vi "send_fpga_config_if_not_imgrid (SubVI).vi"(8 "config_trig":dbl[](array[numeric]) format="%0.2f", 9 "img_cluster":cluster{"Take Pic?":bool, "Only Images":bool}, 10 "file_path_cluster":T2, 11 "channel_settings":T1) -> (3 "Only Images":bool)   [LabVIEW 2022 SP3]
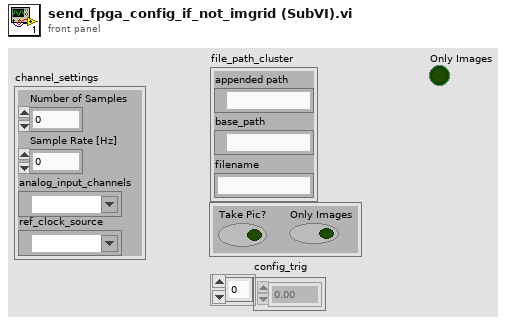
[diagram p1: front panel]
types:
  T1 = cluster{"Number of Samples":i32, "Sample Rate [Hz]":dbl, "analog_input_channels":tag, "ref_clock_source":tag}
  T2 = cluster{"appended path":path, "base_path":path, "filename":string}
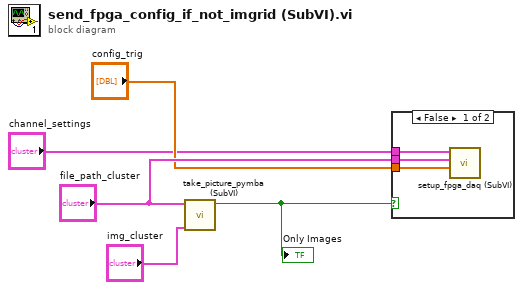
[diagram p0: block diagram]
diagram:
  n1 = call "take_picture_pymba (SubVI).vi"("file_path_cluster"="file_path_cluster", "img_cluster"="img_cluster") -> ("Only Images"=w4:bool)  [unwired: 8 in]
  "Only Images" <- w4
  n2 = case shown="False" w4 {
    tunnel: "channel_settings" -> [w6 _]
    tunnel: "file_path_cluster" -> [w8 _]
    tunnel: "config_trig" -> [w7 _]
    frame False {
      n3 = call "setup_fpga_daq (SubVI).vi"("config_trig"=w7, "file_path_cluster"=w8, "channel_settings"=w6) -> ()  [unwired: 9 in]
    }
    frame True {
    }
  }
